vi "Wrapper.vi"(0 "measurement configuration":T1={"Virtual Device Name"="Lorem ipsum dolor sit", "Option String (\"\")"="", "Connection Specification (\"\")"="", "Disconnection Specification (\"\")"=""}, 11 "error in":errorcluster) -> (4 "measurement results":T2, 15 "error out":errorcluster)   [LabVIEW 2021, in "SimpleSwitch.lvlib"]
uses:
  SimpleSwitch.lvlib
  Measurement Results.ctl
  Measurement Configuration.ctl
  MeasurementCore/SimpleSwitch/SimpleSwitch_Reusables.lvlib
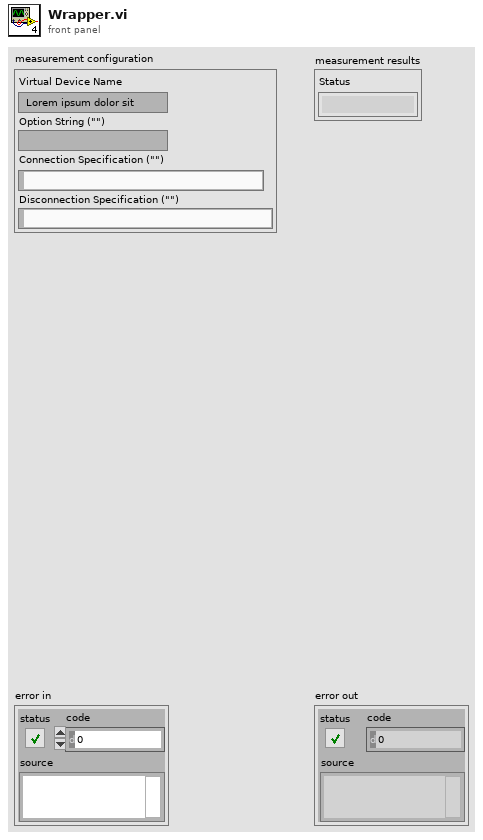
[diagram p1: front panel]
types:
  T1 = typedef "SimpleSwitch.lvlib/Measurement Configuration.ctl" = cluster{"Virtual Device Name":string, "Option String (\"\")":string, "Connection Specification (\"\")":string, "Disconnection Specification (\"\")":string}
  T2 = typedef "SimpleSwitch.lvlib/Measurement Results.ctl" = cluster{"Status":string}
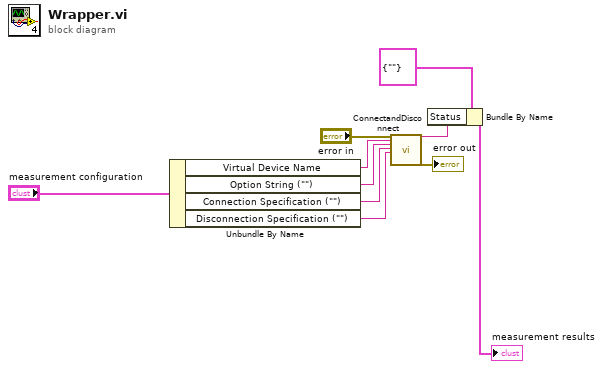
[diagram p0: block diagram]
diagram:
  n1 = Unbundle By Name("measurement configuration") -> ("Virtual Device Name"=w9:string, "Option String (\"\")"=w8:string, "Connection Specification (\"\")"=w7:string, "Disconnection Specification (\"\")"=w6:string)
  n2 = call "ConnectandDisconnect.vi"("error in"="error in", "Virtual Device Name"=w9, "Option String (\"\")"=w8, "Connection Specification (\"\")"=w7, "Disconnection Specification (\"\")"=w6) -> ("Status"=w3:string, "error out"=→"error out":errorcluster)  [unwired: 21 in]
  n3 = Bundle By Name(cluster=T2 {"Status"=""} ("measurement results"), "Status"=w3) -> (→"measurement results":T2)
